vi "Close.vi"(8 "error in (no error)":errorcluster, 11 "uService Template in":refnum<class "Scheduler.lvclass">) -> (0 "error out":errorcluster, 3 "uService Template out":refnum<class "Scheduler.lvclass">)   [LabVIEW 2020, in "TALOS.lvlib" / "Scheduler.lvlib" / "Scheduler.lvclass"]
uses:
  Scheduler.lvclass
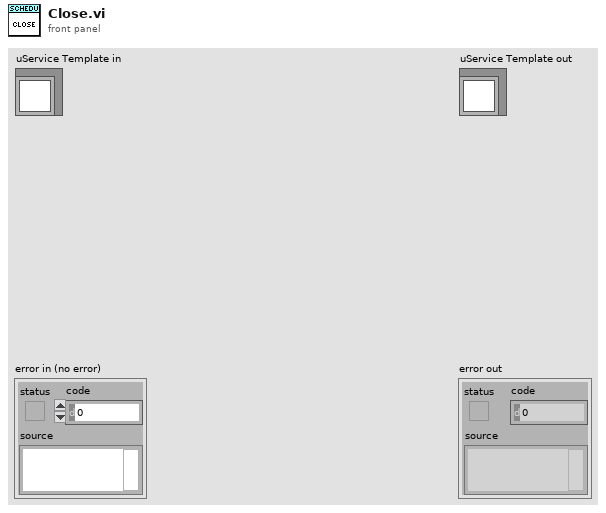
[diagram p1: front panel]
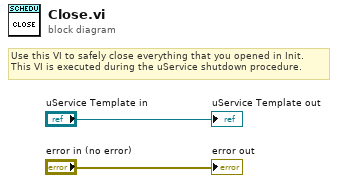
[diagram p0: block diagram]
diagram:
  # "Use this VI to safely close everything that you opened in Init.\nThis VI is executed during the uService shutdown procedure."
  "error out" <- "error in (no error)"
  "uService Template out" <- "uService Template in"
